vi "Read Headers.vi"(8 "error in (no error)":errorcluster, 11 "WebsocketsConnection in":refnum<class "WebsocketsConnection.lvclass">) -> (0 "error out":errorcluster, 2 "Return Headers":variant, 3 "WebsocketsConnection out":refnum<class "WebsocketsConnection.lvclass">)   [LabVIEW 2013, in "MQTT_Websockets.lvlib" / "WebsocketsConnection.lvclass"]
uses:
  WebsocketsConnection.lvclass
  WebsocketsConnection.lvclass/WebsocketsConnection.ctl
  <vilib>/MediaMongrels Ltd/WebSockets/WebSockets/WebSocket/WebSocket.lvclass/WebSocket.ctl
  <vilib>/MediaMongrels Ltd/WebSockets/WebSockets/WebSocket/Read Return Headers.vi
  <vilib>/MediaMongrels Ltd/WebSockets/WebSockets/WebSocket/WebSocket.lvclass
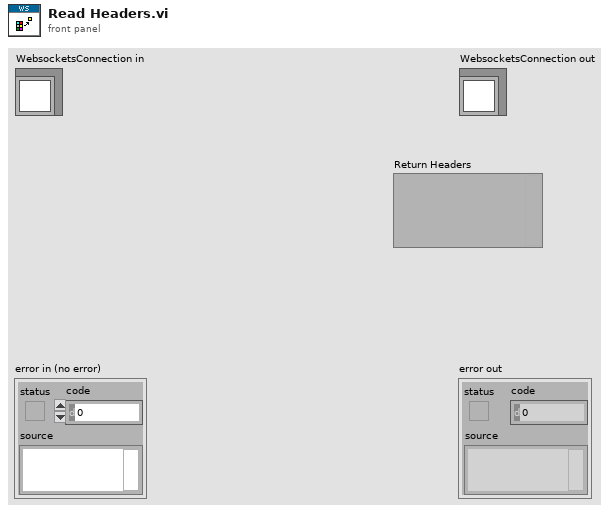
[diagram p1: front panel]
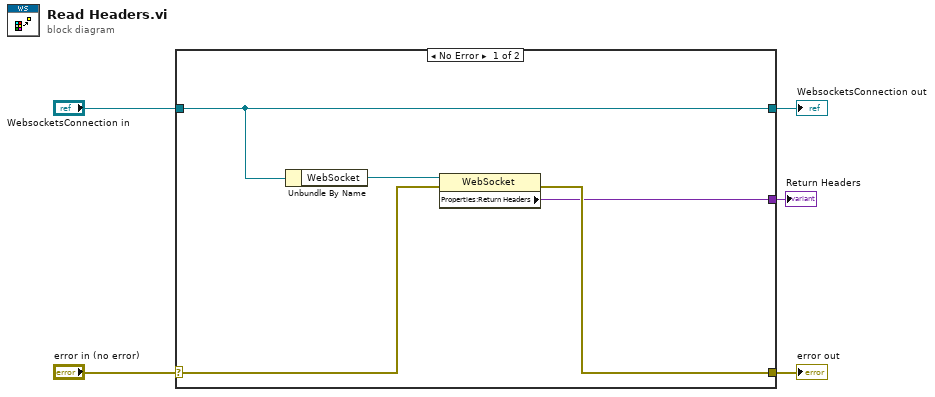
[diagram p0: block diagram]
diagram:
  n1 = case shown="No Error" "error in (no error)" {
    selector: "error in (no error)" -> [w8 w12]
    tunnel: [w7 w12] -> w4
    tunnel: [w10 w11] -> w2
    tunnel: "WebsocketsConnection in" -> [w10 w11]
    tunnel: [w6 _] -> w1
    frame No Error {
      n2 = Unbundle By Name(w10) -> ("WebSocket"=w9:refnum<class "WebSocket.lvclass">)
      n3 = property class="WebSocket"(reference=w9, error in=w8) -> (error out=w7:errorcluster, "Properties:Return Headers"=w6:variant)  [unwired: 1 out]
    }
    frame Error {
    }
  }
  "error out" <- w4
  "WebsocketsConnection out" <- w2
  "Return Headers" <- w1
